vi "closeDocument.vi"(8 "error in (no error)":errorcluster, 11 "workbook in":refnum<class "workbook.lvclass">) -> (0 "error out":errorcluster, 3 "workbook out":refnum<class "workbook.lvclass">)   [LabVIEW 2017, in "Excel_Specific.lvlib" / "workbook.lvclass"]
uses:
  workbook.lvclass
  workbook.lvclass/workbook.ctl
  worksheet/worksheet.lvclass
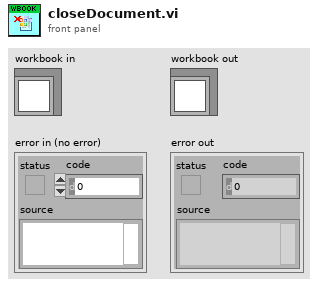
[diagram p1: front panel]
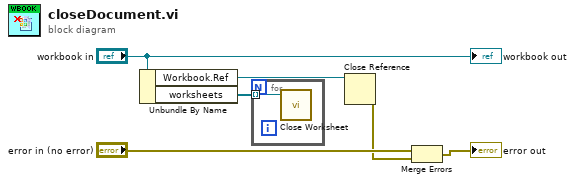
[diagram p0: block diagram]
diagram:
  n1 = Unbundle By Name("workbook in") -> ("Workbook.Ref"=w4:refnum<k24>, "worksheets"=w1:refnum<class "worksheet.lvclass">[])
  n2 = for {
    tunnel: w1 -> [w7] mode=indexing
    n3 = call "Close Worksheet.vi"("worksheet in"=w7) -> ()  [unwired: 9 in, 2 out]
  }
  n4 = Close Reference(reference=w4) -> (error out=w2:errorcluster)  [unwired: 1 in]
  n5 = Merge Errors("error in (no error)", w2) -> (→"error out":errorcluster)
  "workbook out" <- "workbook in"
